vi "initialize multimeter.vi"(6 "trigger mode (0:internal)":u16(ring) items=["internal - continuous trigger", "external - rear panel trigger with delay", "external - bus trigger with delay", "external - rear panel trigger", "external - bus trigger"], 7 "function (0:volts DC)":u16(ring) items=["volts DC", "volts AC", "2-wire k.ohms", "4-wire k.ohms", "mA DC", "mA AC"], 8 "error in (no error)":errorcluster, 9 "rate (0:slow)":u16(ring)=2 items=["slow", "medium", "fast"], 10 "range (0:auto)":u16(ring) items=["autorange", "200mV, 200 ohms", "2V, 2 kohms", "20V, 20 kohms", "200V, 200 kohms", "1000Vdc, 700 Vac, 2 Mohms", "20 Mohms"], 11 "VISA resource name":refnum<visa-resource-name>="GPIB0::2::INSTR") -> (0 "error out":errorcluster, 1 "unit":string, 2 "measurement":dbl format="%^.6e", 3 "VISA resource name out":refnum<visa-resource-name>)   [LabVIEW 2012, in "Varian.lvlib"]
doc: "The Application Example configures, triggers and reads back the measurement from the Fluke 8840A and the Fluke 8842A digital multimeters. The configuration subVI used is for the 8840A, but it works on the 8842A as well. The only difference in the two configure VIs is that the FL8842A Configure has one more optional range setting than the FL8840A."
uses:
  Varian.lvlib
  Fluke Multimeter/Fluke 8840/Fluke 8840.lvlib
panel:
  # "Copyright 2005. National Instruments Corporation."
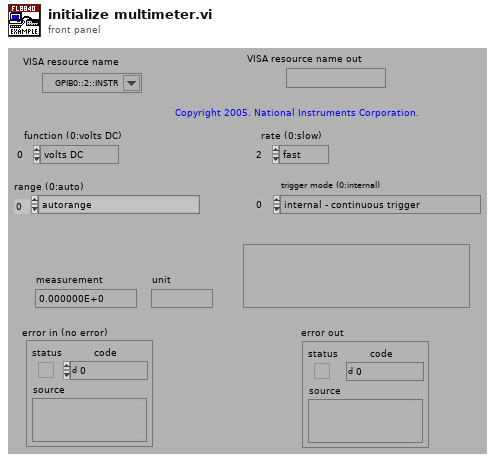
[diagram p1: front panel]
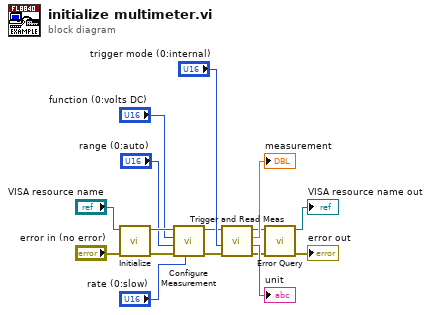
[diagram p0: block diagram]
diagram:
  n1 = call "Initialize.vi"("error in (no error)"="error in (no error)", "VISA resource name"="VISA resource name") -> ("error out"=w6:errorcluster, "VISA resource name out"=w5:refnum<visa-resource-name>)  [unwired: 1 in, 7 out]
  n2 = call "Configure Measurement.vi"("rate (0:slow)"="rate (0:slow)", "error in (no error)"=w6, "range (0:auto)"="range (0:auto)", "function (0:volts DC)"="function (0:volts DC)", "VISA resource name"=w5) -> ("error out"=w8:errorcluster, "VISA resource name out"=w7:refnum<visa-resource-name>)  [unwired: 5 out]
  n3 = call "Trigger and Read Meas.vi"("error in (no error)"=w8, "trigger mode (0:internal)"="trigger mode (0:internal)", "VISA resource name"=w7) -> ("error out"=w9:errorcluster, "unit"=→"unit":string, "measurement"=→"measurement":dbl, "VISA resource name out"=w11:refnum<visa-resource-name>)  [unwired: 5 out]
  n4 = call "Error Query.vi"("error in (no error)"=w9, "VISA resource name"=w11) -> ("error out"=→"error out":errorcluster, "VISA resource name out"=→"VISA resource name out":refnum<visa-resource-name>)  [unwired: 1 in, 7 out]
